vi "Set_Rescaling_Setting.vi"(6 "isOriginalMonitor":bool, 8 "error in (no error)":errorcluster, 9 "avg":dbl, 10 "mode":i32(ring) items=["Freerun_SPU", "Freerun_Referencemodule"], 11 ".NET Reference in":refnum<k24>) -> (0 "error out":errorcluster, 3 "Reference out":refnum<k24>)   [LabVIEW 2017]
doc: "Setting for STS rescaling mode"
uses:
  D:/test/PDLSTS/LV_PDL_Sample/DLL/STSProcess.dll
  DLL/STSProcess.dll
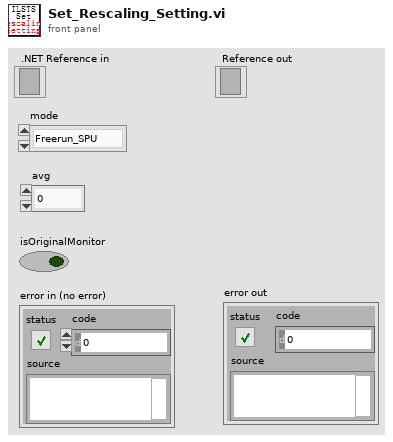
[diagram p1: front panel]
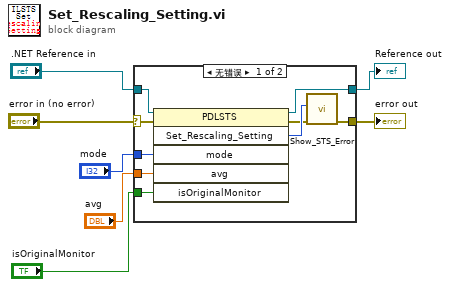
[diagram p0: block diagram]
diagram:
  n1 = case shown="无错误" "error in (no error)" {
    selector: "error in (no error)" -> [w14 w18]
    tunnel: ".NET Reference in" -> [w16 w17]
    tunnel: [w15 w17] -> w6
    tunnel: [w11 w18] -> w4
    tunnel: "mode" -> [w10 _]
    tunnel: "avg" -> [w9 _]
    tunnel: "isOriginalMonitor" -> [w8 _]
    frame No Error {
      n2 = invoke on="调用节点" class="PDLSTS" method="Set_Rescaling_Setting"(reference=w16, error in=w14, "mode"=w10, "avg"=w9, "isOriginalMonitor"=w8) -> (reference out=w15:refnum<k24>, error out=w12:errorcluster, "Set_Rescaling_Setting"=w13:i32)  [unwired: 1 in, 3 out]
      n3 = call "Show_STS_Error.vi"("error in (no error)"=w12, "Error"=w13) -> ("error out"=w11:errorcluster)  [unwired: 9 in]
    }
    frame Error {
    }
  }
  "error out" <- w4
  "Reference out" <- w6
